vi "ProcessWithOutput.vi"() -> ()   [LabVIEW 2013]
uses:
  <vilib>/Instr/_visa.llb/VISA Configure Serial Port (Instr).vi
panel:
  in  "Serial Output":refnum<visa-resource-name>="COM9"
  out "Stellwinkel":dbl(knob)=-28.514851485148544 scale=-90.0..90.0
  in  "Winkel des Hauses zum Spiegel":dbl(knob) scale=-90.0..90.0
  out "Standardabweichung":dbl=3.954535892818606
  out "Ready":bool=TRUE
  out "Line Received":bool
  in  "Serial Input":refnum<visa-resource-name>="COM5"
  in  "Smoothing":bool
  out "Einfallswinkel":dbl(knob)=-30.0 scale=-90.0..90.0
  in  "Gaussian Fit":bool=TRUE
  in  "Stop Button":bool=TRUE
  # "Osten"
  # "Westen"
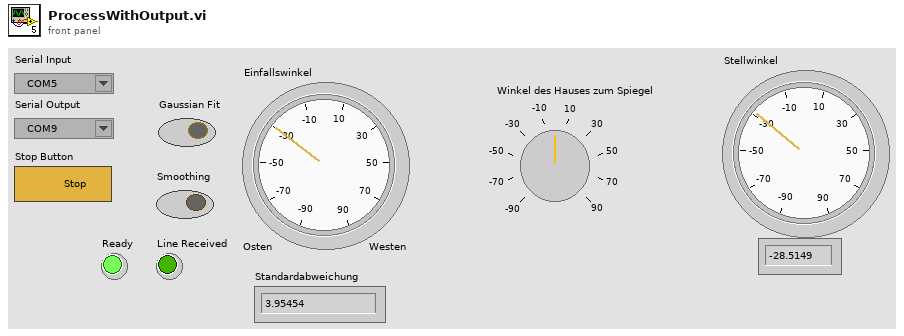
[diagram p1: front panel]
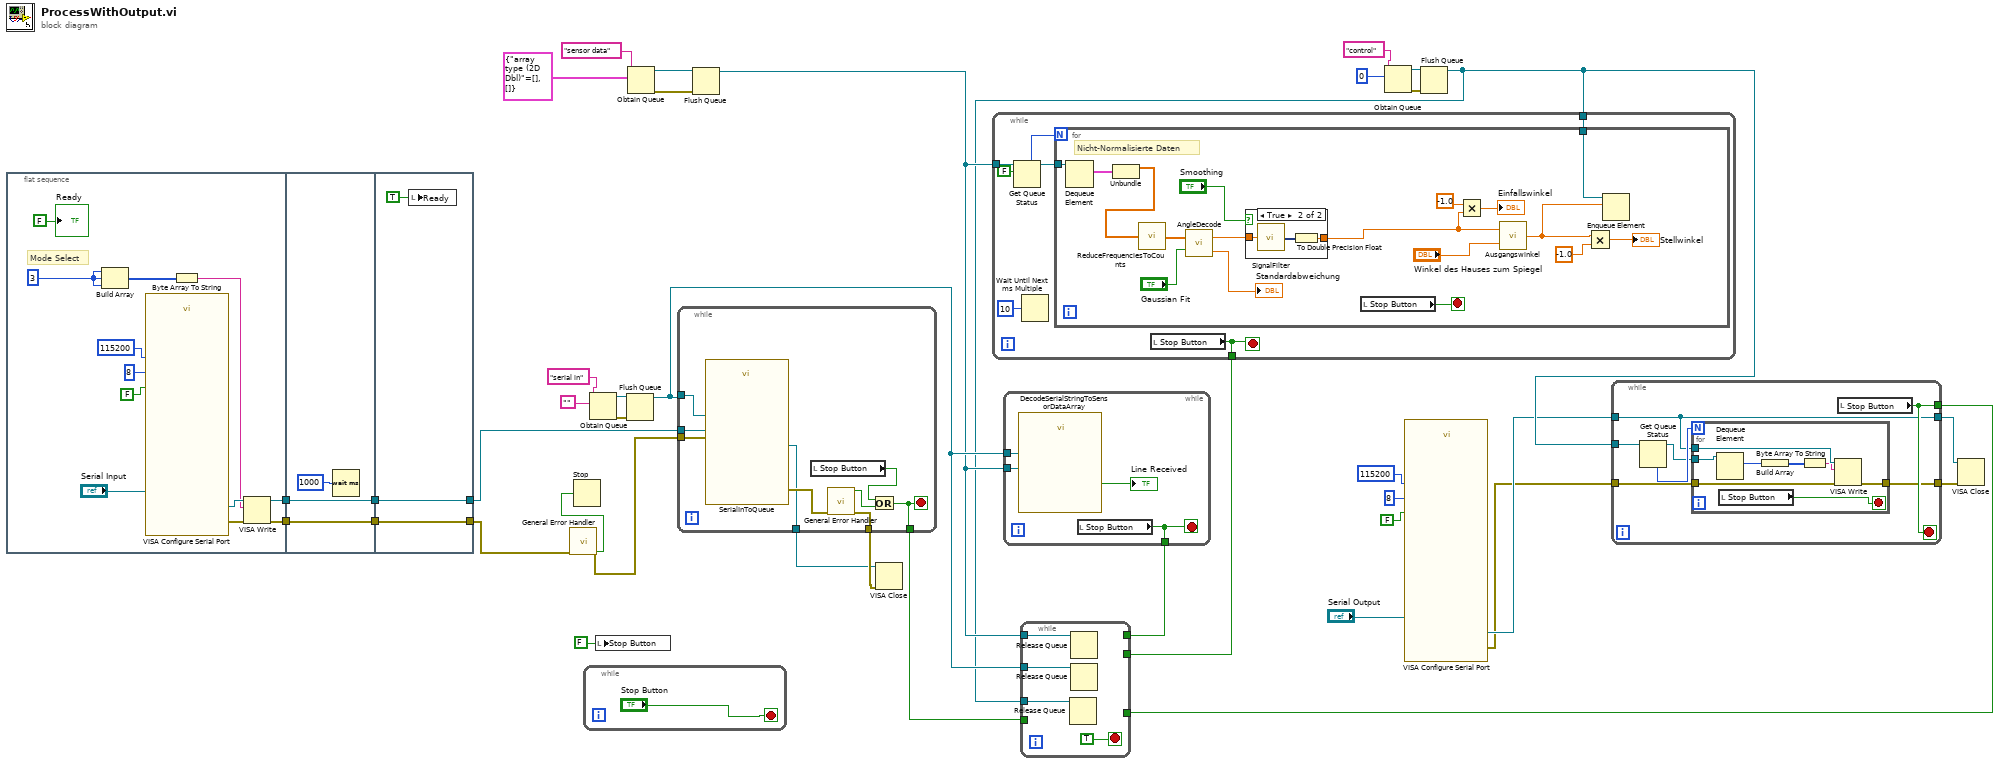
[diagram p0: block diagram]
diagram:
  n1 = flat-sequence {
    tunnel: [w43] -> w16
    tunnel: [w42] -> w15
    tunnel: [w52] -> w18
    tunnel: [w51] -> w17
    tunnel: w16 -> [w52]
    tunnel: w15 -> [w51]
    tunnel: [w54] -> w19
    tunnel: [w55] -> w20
    tunnel: w18 -> [w55]
    tunnel: w17 -> [w54]
    frame #0 {
      w45 = u8 3 ("number")
      # "Mode Select"
      n2 = Build Array(w45, w45, w45) -> (w46:u8[])
      n3 = call-poly "VISA Configure Serial Port"("VISA resource name"="Serial Input", "Enable Termination\nChar (T)"=FALSE ("Enable Termination\nChar (T)"), "baud rate (9600)"=u32 115200, "data bits (8)"=u16 8) -> ("VISA resource name out"=w41:refnum<visa-resource-name>, "error out"=w40:errorcluster)  [unwired: 10 in]
      n4 = Byte Array To String(unsigned byte array=w46) -> (string=w39:string)
      n5 = VISA Write(VISA resource name=w41, write buffer=w39, error in (no error)=w40) -> (VISA resource name out=w43:refnum<visa-resource-name>, error out=w42:errorcluster)  [unwired: 1 out]
      "Ready" <- FALSE ("Ready")
    }
    frame #1 {
      n6 = Wait (ms)(milliseconds to wait=u32 1000) -> ()  [unwired: 1 out]
    }
    frame #2 {
      n7 = local write "Ready"(TRUE ("Ready")) -> ()
    }
  }
  n8 = call <vilib>:"General Error Handler.vi"("error in (no error)"=w19) -> ("error?"=w29:bool, "error out"=w30:errorcluster)  [unwired: 10 in, 3 out]
  n9 = Stop(stop? (T)=w29) -> ()
  n10 = while {
    stop <- "Stop Button" stop-if-true
  }
  n11 = Obtain Queue(name (unnamed)="serial in", element data type="") -> (queue out=w32:refnum<queue>, error out=w31:errorcluster)  [unwired: 3 in, 1 out]
  n12 = local write "Stop Button"(FALSE ("Stop Button")) -> ()
  n13 = Flush Queue(queue=w32, error in (no error)=w31) -> (queue out=w26:refnum<queue>)  [unwired: 2 out]
  n14 = Obtain Queue(name (unnamed)="sensor data", element data type=cluster{"array type (2D Dbl)":dbl[], dbl[]} {"array type (2D Dbl)"=[], []} ("output cluster")) -> (queue out=w34:refnum<queue>, error out=w33:errorcluster)  [unwired: 3 in, 1 out]
  n15 = while {
    tunnel: w20 -> [w66]
    tunnel: w26 -> [w60]
    tunnel: w30 -> [w65]
    tunnel: [w64] -> w28
    tunnel: [w59] -> w24
    tunnel: [w58] -> w21
    stop <- w59 stop-if-true
    n16 = call "SerialInToQueue.vi"("error in (no error)"=w65, "VISA resource name in"=w66, "Queue in"=w60) -> ("error out"=w63:errorcluster, "VISA resource name"=w58:refnum<visa-resource-name>)  [unwired: 5 in, 2 out]
    n17 = local read "Stop Button"() -> (w61:bool)
    n18 = call <vilib>:"General Error Handler.vi"("error in (no error)"=w63) -> ("error?"=w62:bool, "error out"=w64:errorcluster)  [unwired: 10 in, 3 out]
    n19 = Or(x=w61, y=w62) -> (x .or. y?=w59:bool)
  }
  n20 = Flush Queue(queue=w34, error in (no error)=w33) -> (queue out=w25:refnum<queue>)  [unwired: 2 out]
  n21 = VISA Close(VISA resource name=w21, error in (no error)=w28) -> ()  [unwired: 1 out]
  n22 = while {
    tunnel: w25 -> [w70]
    tunnel: w26 -> [w68]
    tunnel: [w67] -> w23
    stop <- w67 stop-if-true
    n23 = call "DecodeSerialStringToSensorDataArray.vi"("Serial String Queue in"=w68, "Sensor Data Queue in"=w70) -> ("Line Received"=→"Line Received":bool)  [unwired: 1 out]
    n24 = local read "Stop Button"() -> (w67:bool)
  }
  n25 = Obtain Queue(name (unnamed)="control", element data type=i8 0) -> (queue out=w13:refnum<queue>, error out=w12:errorcluster)  [unwired: 3 in, 1 out]
  n26 = call-poly "VISA Configure Serial Port"("VISA resource name"="Serial Output", "Enable Termination\nChar (T)"=FALSE ("Enable Termination\nChar (T)"), "baud rate (9600)"=u32 115200, "data bits (8)"=u16 8) -> ("VISA resource name out"=w3:refnum<visa-resource-name>, "error out"=w2:errorcluster)  [unwired: 10 in]
  n27 = Flush Queue(queue=w13, error in (no error)=w12) -> (queue out=w9:refnum<queue>)  [unwired: 2 out]
  n28 = while {
    tunnel: w25 -> [w76]
    tunnel: [w75] -> w22
    tunnel: w9 -> [w72]
    stop <- w75 stop-if-true
    n29 = Get Queue Status(queue=w76, return elements? (F)=FALSE) -> (queue out=w73:refnum<queue>, # elements in queue=w77:i32)  [unwired: 1 in, 6 out]
    n30 = Wait Until Next ms Multiple(millisecond multiple=u32 10) -> ()  [unwired: 1 out]
    n31 = for {
      N: w77 -> [_]
      tunnel: w73 -> [w89]
      tunnel: w72 -> [w85]
      stop <- w90 stop-if-true
      # "Nicht-Normalisierte Daten"
      n32 = Dequeue Element(queue=w89) -> (element=w88:cluster{"array type (2D Dbl)":dbl[], dbl[]})  [unwired: 2 in, 3 out]
      n33 = Unbundle(w88) -> ("array type (2D Dbl)"=w91:dbl[])  [unwired: 1 out]
      n34 = call "ReduceFrequenciesToCounts.vi"("Sensor Frequencies (kHz)"=w91) -> ("Sensor Counts"=w92:dbl[])
      n35 = call "AngleDecode.vi"("Interpolate"="Gaussian Fit", "Data"=w92) -> ("Standard Deviation"=→"Standardabweichung":dbl, "Peak Angle"=w94:dbl)
      n36 = case shown="True" "Smoothing" {
        tunnel: w94 -> [w95 w98]
        tunnel: [w95 w96] -> w81
        frame False {
        }
        frame True {
          n37 = call "SignalFilter.vi"("Signal In"=w98) -> ("Filtered Signal"=w97:dynamicdata)
          n38 = To Double Precision Float(number=w97) -> (double precision float=w96:dbl)
        }
      }
      n39 = local read "Stop Button"() -> (w90:bool)
      n40 = Multiply(x=-1.0 ("y"), y=w81) -> (x*y=→"Einfallswinkel":dbl)
      n41 = call "Ausgangswinkel.vi"("Hauswinkel"="Winkel des Hauses zum Spiegel", "Einfallswinkel"=w81) -> ("Stellwinkel"=w79:dbl)
      n42 = Multiply(x=w79, y=-1.0) -> (x*y=→"Stellwinkel":dbl)
      n43 = Enqueue Element(queue=w85, element=w79) -> ()  [unwired: 2 in, 3 out]
    }
    n44 = local read "Stop Button"() -> (w75:bool)
  }
  n45 = while {
    tunnel: [w105] -> w10
    tunnel: w9 -> [w104]
    tunnel: [w101] -> w4
    tunnel: w3 -> [w101]
    tunnel: [w99] -> w1
    tunnel: w2 -> [w100]
    stop <- w105 stop-if-true
    n46 = Get Queue Status(queue=w104) -> (queue out=w102:refnum<queue>, # elements in queue=w103:i32)  [unwired: 2 in, 6 out]
    n47 = for {
      N: w103 -> [_]
      tunnel: w102 -> [w112]
      tunnel: w101 -> [w110]
      tunnel: w100 -> [w109]
      tunnel: [w108] -> w99
      stop <- w106 stop-if-true
      n48 = Dequeue Element(queue=w112) -> (element=w111:i8)  [unwired: 2 in, 3 out]
      n49 = local read "Stop Button"() -> (w106:bool)
      n50 = Build Array(w111) -> (w113:i8[])
      n51 = Byte Array To String(unsigned byte array=w113) -> (string=w107:string)
      n52 = VISA Write(VISA resource name=w110, write buffer=w107, error in (no error)=w109) -> (error out=w108:errorcluster)  [unwired: 2 out]
    }
    n53 = local read "Stop Button"() -> (w105:bool)
  }
  n54 = while {
    tunnel: w26 -> [w116]
    tunnel: w25 -> [w115]
    tunnel: w24 -> [_]
    tunnel: w23 -> [_]
    tunnel: w22 -> [_]
    tunnel: w9 -> [w114]
    tunnel: w10 -> [_]
    stop <- TRUE stop-if-true
    n55 = Release Queue(queue=w114) -> ()  [unwired: 2 in, 3 out]
    n56 = Release Queue(queue=w115) -> ()  [unwired: 2 in, 3 out]
    n57 = Release Queue(queue=w116) -> ()  [unwired: 2 in, 3 out]
  }
  n58 = VISA Close(VISA resource name=w4, error in (no error)=w1) -> ()  [unwired: 1 out]
